vi "csm-lv-project.vi"() -> ()   [LabVIEW 2017, in "testcase-miscellaneous.lvclass"]
uses:
  testcase-miscellaneous.lvclass
  src/project/Communicable State Machine(CSM)/csm_tool_menu.lvlib
  src/user.lib/_NEVSTOP/Communicable State Machine(CSM)/_tool/_ui/csm-ui-support.lvlib
panel:
  out "error out":errorcluster
  in  "error in (no error)":errorcluster
  in  "VI Ref":refnum<vi>
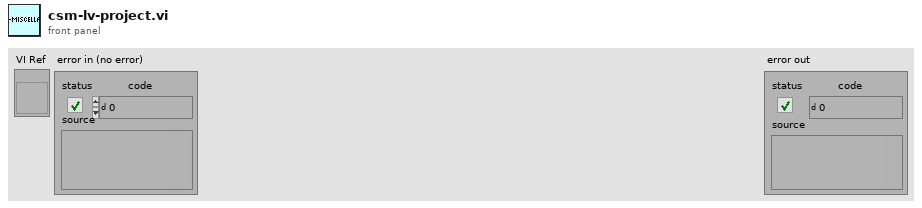
[diagram p1: front panel]
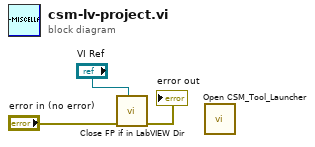
[diagram p0: block diagram]
diagram:
  n1 = call "Close FP if in LabVIEW Dir.vi"("VI Refnum"="VI Ref", "Error in"="error in (no error)") -> ("Error out"=→"error out":errorcluster)  [unwired: 9 in]
  n2 = call "Open CSM_Tool_Launcher.vi"() -> ()  [unwired: 12 in]
